vi "(SubVI)_2Dsave_bin_BD_Ver6.vi"(8 "Error In":errorcluster, 9 "Number of B-scans":i32, 10 "refnum in":refnum<file>, 11 "queue in":refnum<queue>) -> (0 "error out":errorcluster, 2 "double precision float":dbl, 3 "prepend array or string size? (T)":bool)   [LabVIEW 2019]
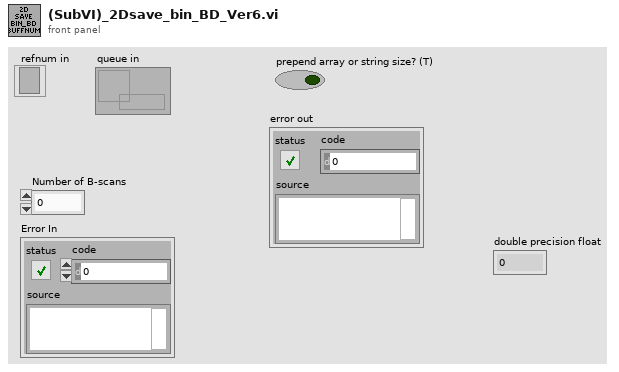
[diagram p1: front panel]
types:
  T1 = enum16{"big-endian, network order", "native, host order", "little-endian"}
  T2 = cluster{"Image Pixels (I16)":i16[][], "double precision float":dbl}
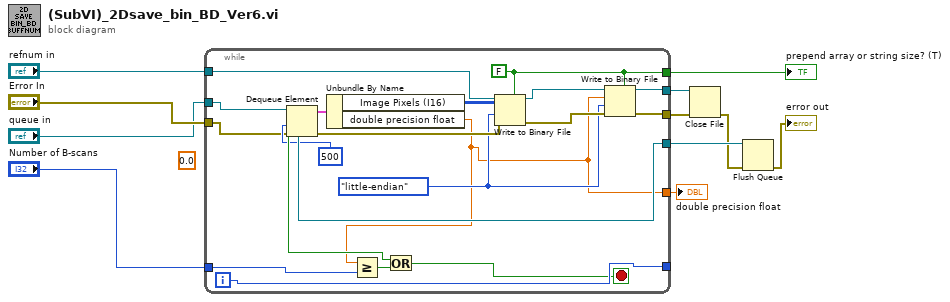
[diagram p0: block diagram]
diagram:
  (unwired) 0.0 ("double precision float")
  n1 = while {
    tunnel: "queue in" -> [w13]
    tunnel: "Error In" -> [w12]
    tunnel: "refnum in" -> [w25]
    tunnel: [w22] -> w8
    tunnel: [w30] -> w11
    tunnel: "Number of B-scans" -> [w29]
    tunnel: [w19] -> w6
    tunnel: [w18] -> w5
    tunnel: [w14] -> w1
    tunnel: [w16] -> _
    i -> [w16]
    stop <- w15 stop-if-true
    w23 = T1."little-endian" ("byte order (0:big-endian, network order)")
    w22 = FALSE ("prepend array or string size? (T)")
    n2 = Dequeue Element(queue=w13, timeout in ms (-1)=500, error in (no error)=w12) -> (queue out=w30:refnum<queue>, element=w21:T2, timed out?=w27:bool, error out=w31:errorcluster)
    n3 = Unbundle By Name(w21) -> ("Image Pixels (I16)"=w20:i16[][], "double precision float"=w14:dbl)
    n4 = Greater Or Equal?(x=w14, y=w29) -> (x >= y?=w28:bool)
    n5 = Or(x=w27, y=w28) -> (x .or. y?=w15:bool)
    n6 = Write to Binary File(file (use dialog)=w25, data=w20, error in=w31, 5:w22, 9:w23) -> (refnum out=w24:refnum<file>, error out=w26:errorcluster)  [unwired: 1 in, 1 out]
    n7 = Write to Binary File(file (use dialog)=w24, data=w14, error in=w26, 5:w22, 9:w23) -> (refnum out=w18:refnum<file>, error out=w19:errorcluster)  [unwired: 1 in, 1 out]
  }
  "prepend array or string size? (T)" <- w8
  "double precision float" <- w1
  n8 = Close File(refnum=w5, error in=w6) -> (error out=w9:errorcluster)  [unwired: 1 out]
  n9 = Flush Queue(queue=w11, error in (no error)=w9) -> (error out=→"error out":errorcluster)  [unwired: 2 out]
